vi "NumToDigits(U64).vi"(8 "error in (no error)":errorcluster caption="错误输入（无错误）", 10 "基数 (10)":u64=10, 11 "输入数值":u64) -> (0 "error out":errorcluster caption="错误输出", 2 "总位数":i32, 3 "位数数组":u64[](array[numeric]))   [LabVIEW 2012]
doc: "Converts a single I32 into an array of digits, in order of increasing significance. If the input number is negative, the most significant digit (last element of the array) is also negative. All other digits are always non-negative. By default, the output digits are the digits used to represent the number in base 10, though the base can be changed. For example, the binary representation can be obtained by wiring the value 2 to the Base input. Note that Base is coerced to a minimum value of 2.\n\nAs long as no coersion is required, the original number can be recreated as\nN = Digits[0] * Base^0 + Digits[1] * Base^1 + Digits[2] * Base^2 + ... + Digits[n] * Base^n\n\nFreeware from Moore Good Ideas, www.mooregoodideas.com. Do not remove this line."
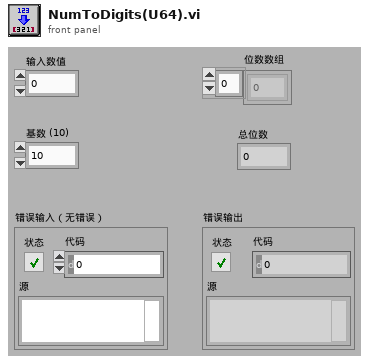
[diagram p1: front panel]
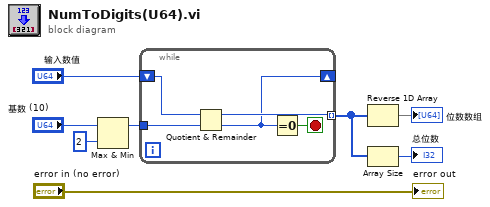
[diagram p0: block diagram]
diagram:
  n1 = Max & Min(x="基数 (10)", y=u64 2) -> (max(x,y)=w7:u64)  [unwired: 1 out]
  n2 = while {
    tunnel: w7 -> [w13]
    tunnel: [w11] -> w2 mode=indexing
    shift-right: [w9] -> _
    shift-left: "输入数值" -> [w10]
    stop <- w12 stop-if-true
    n3 = Quotient & Remainder(x=w10, y=w13) -> (x-y*floor(x/y)=w11:u64, floor(x/y)=w9:u64)
    n4 = Equal To 0?(x=w9) -> (x = 0?=w12:bool)
  }
  n5 = Reverse 1D Array(array=w2) -> (reversed array=→"位数数组":u64[])
  n6 = Array Size(array=w2) -> (size(s)=→"总位数":i32)
  "error out" <- "error in (no error)"
